vi "Type.vi"(11 "TextPanel in":refnum<class "TextPanel.lvclass">) -> (2 "Type":refnum<class "Type.lvclass">)   [LabVIEW 2020, in "Conditum-Tools.lvlib" / "TextPanel.lvclass"]
uses:
  TextPanel.lvclass
  Conditum-Clone/Columns/Type/Type.lvclass
  Conditum-Clone/Columns/Text/Text.lvclass
  C:/dev/lv20CE/lv-conditum-tools/Conditum-Clone/Columns/Type/Type.lvclass
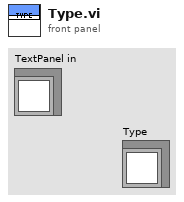
[diagram p1: front panel]
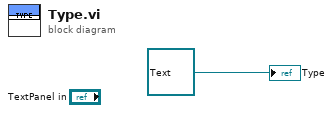
[diagram p0: block diagram]
diagram:
  "Type" <- refnum<class "Text.lvclass"> refnum ("Conditum:Columns:Text.lvclass")
